vi "Generate Method Description.vi"(7 "Name":string, 9 "Status":T1, 10 "Descirption":string, 11 "Test Tree In":refnum<class "Test Result Tree V2.lvclass">) -> (2 "Description":string, 3 "Test Tree Out":refnum<class "Test Result Tree V2.lvclass">)   [LabVIEW 2020, in "Test Result Tree V2.lvclass"]
uses:
  Test Result Tree/Test Result Tree V2.lvclass
  Result/Status.ctl
  Test Result Tree/Test Result Tree V2.lvclass/Test Result Tree V2.ctl
  Test Result Tree Test/Private/Counter Map Key.ctl
  Result/Result.lvlib
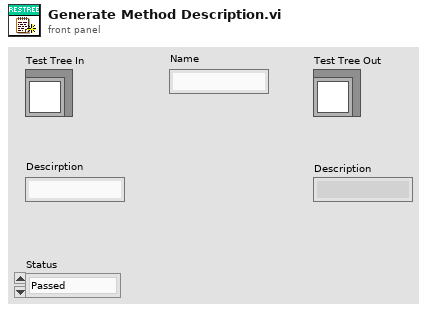
[diagram p1: front panel]
types:
  T1 = typedef "Result.lvlib/Status.ctl" = enum16{"Passed", "Failed", "Error", "Skipped", "Setup Error", "Broken", "Teardown Error"}
  T2 = typedef "Test Result Tree V2.lvclass/Counter Map Key.ctl" = cluster{"Test Case":string, "Status":T1}
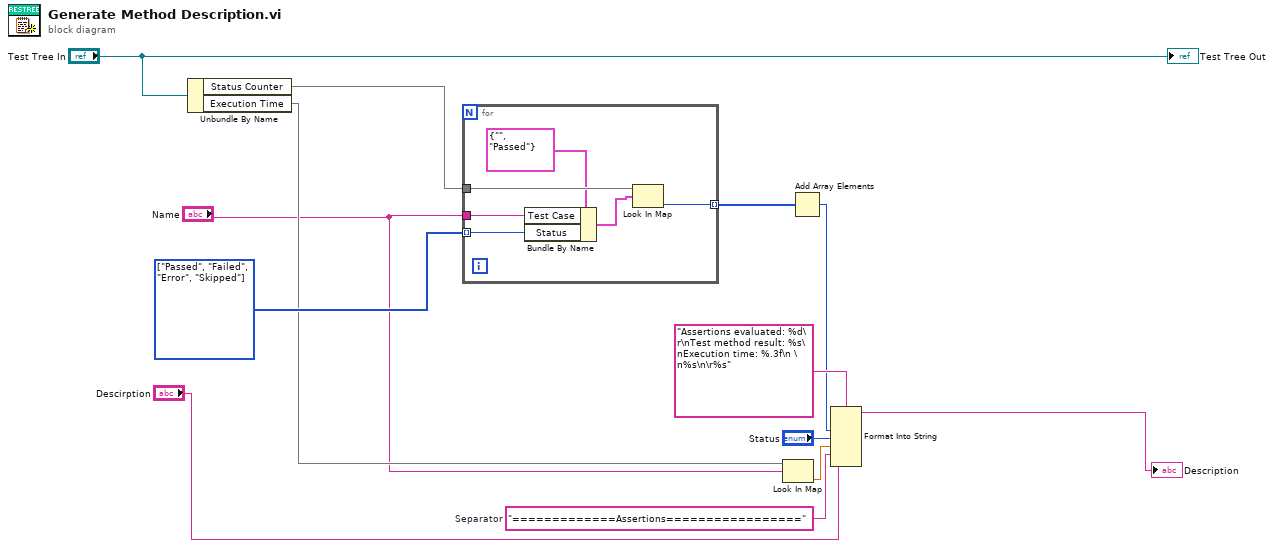
[diagram p0: block diagram]
diagram:
  w7 = T1[] [enum."Passed", enum."Failed", enum."Error", enum."Skipped"] items=["Passed", "Failed", "Error", "Skipped", "Setup Error", "Broken", "Teardown Error"] ("Array")
  w11 = "=============Assertions================="  # Separator
  n1 = Unbundle By Name("Test Tree In") -> ("Status Counter"=w8:map{T2, i32}, "Execution Time"=w3:map{string, dbl})
  n2 = for {
    tunnel: w8 -> [w19]
    tunnel: "Name" -> [w16]
    tunnel: w7 -> [w15] mode=indexing
    tunnel: [w14] -> w6 mode=indexing
    n3 = Bundle By Name(cluster=T2 {"Test Case"="", "Status"=enum."Passed"} ("key"), "Test Case"=w16, "Status"=w15) -> (w17:T2)
    n4 = Look In Map(map=w19, key=w17) -> (value=w14:i32)  [unwired: 1 in, 1 out]
  }
  n5 = Look In Map(map=w3, key="Name") -> (value=w1:dbl)  [unwired: 1 in, 1 out]
  n6 = Add Array Elements(numeric array=w6) -> (sum=w5:i32)
  n7 = Format Into String(format string="Assertions evaluated: %d\r\nTest method result: %s\nExecution time: %.3f\n \n%s\n\r%s", w5, "Status", w1, w11, "Descirption") -> (resulting string=→"Description":string)  [unwired: 2 in, 1 out]
  "Test Tree Out" <- "Test Tree In"
